vi "Engine-DI.vi"(8 "Error In":errorcluster, 11 "DSI Reference":refnum<class "DCM-DSI.lvclass">) -> (0 "Error Out":errorcluster, 3 "DSI Reference":refnum<class "DCM-DSI.lvclass">)   [LabVIEW 2016, in "DSI-RT.lvlib"]
uses:
  DSI-RT.lvlib
  Classes/DCM-DSI/DCM-DSI.lvclass
  <vilib>/addons/Software Calibration Management/xSCM/CalPoint.xnode
  <vilib>/addons/Software Calibration Management/xSCM/ni_scm.dll
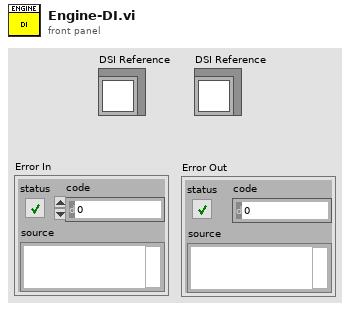
[diagram p1: front panel]
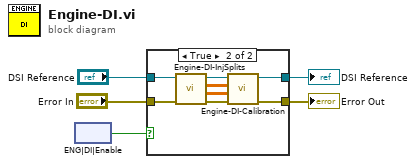
[diagram p0: block diagram]
diagram:
  n1 = xnode "ENG|DI|Enable"() -> ("Value"=w1:bool)
  n2 = case shown="True" w1 {
    tunnel: "DSI Reference" -> [w7 w15]
    tunnel: [w7 w11] -> w4
    tunnel: [w6 w10] -> w3
    tunnel: "Error In" -> [w6 w14]
    frame False {
    }
    frame True {
      n3 = call "Engine-DI-InjSplits.vi"("error in (no error)"=w14, "DCM-DSI.lvclass"=w15) -> ("error out"=w13:errorcluster, "Inj Qtys DI-B"=w8:sgl[][], "Inj Qtys DI-A"=w9:sgl[][], "DCM-DSI.lvclass"=w12:refnum<class "DCM-DSI.lvclass">)  [unwired: 6 in]
      n4 = call "Engine-DI-Calibration.vi"("error in (no error)"=w13, "Inj Qtys DI-B"=w8, "Inj Qtys DI-A"=w9, "DCM DSI"=w12) -> ("error out"=w10:errorcluster, "DCM DSI"=w11:refnum<class "DCM-DSI.lvclass">)  [unwired: 6 in]
    }
  }
  "Error Out" <- w3
  "DSI Reference" <- w4
